vi "Test_Fitting.vi"() -> ()   [LabVIEW 2015]
panel:
  out "best fit parameters":dbl[](array[numeric])=[97.36526335937096, 65.50408984686088, 41.15888694388816, 22.4726351042886, 37.87775155788913]
  out "Generated Image":dbl[][](graph)
  out "error out":errorcluster
  out "Elapsed time in ms":u32=1425
  out "Best Fit":dbl[][](graph)
  in  "Image Size":cluster{"Width":dbl, "Height":dbl}={"Width"=100.0, "Height"=100.0}
  in  "Noise":dbl=10.0
  in  "Simulation":dbl[](array[slide])=[97.19626168224299, 65.42056074766354, 41.1214953271028, 22.429906542056074, 38.006230529595015, 104.04984423676012] caption="Amplitude\n\n\nX-Position\n\n\nY-Position\n\n\nWidth A\n\n\nWidth B\n\n\nAngle" scale=0.0..200.0
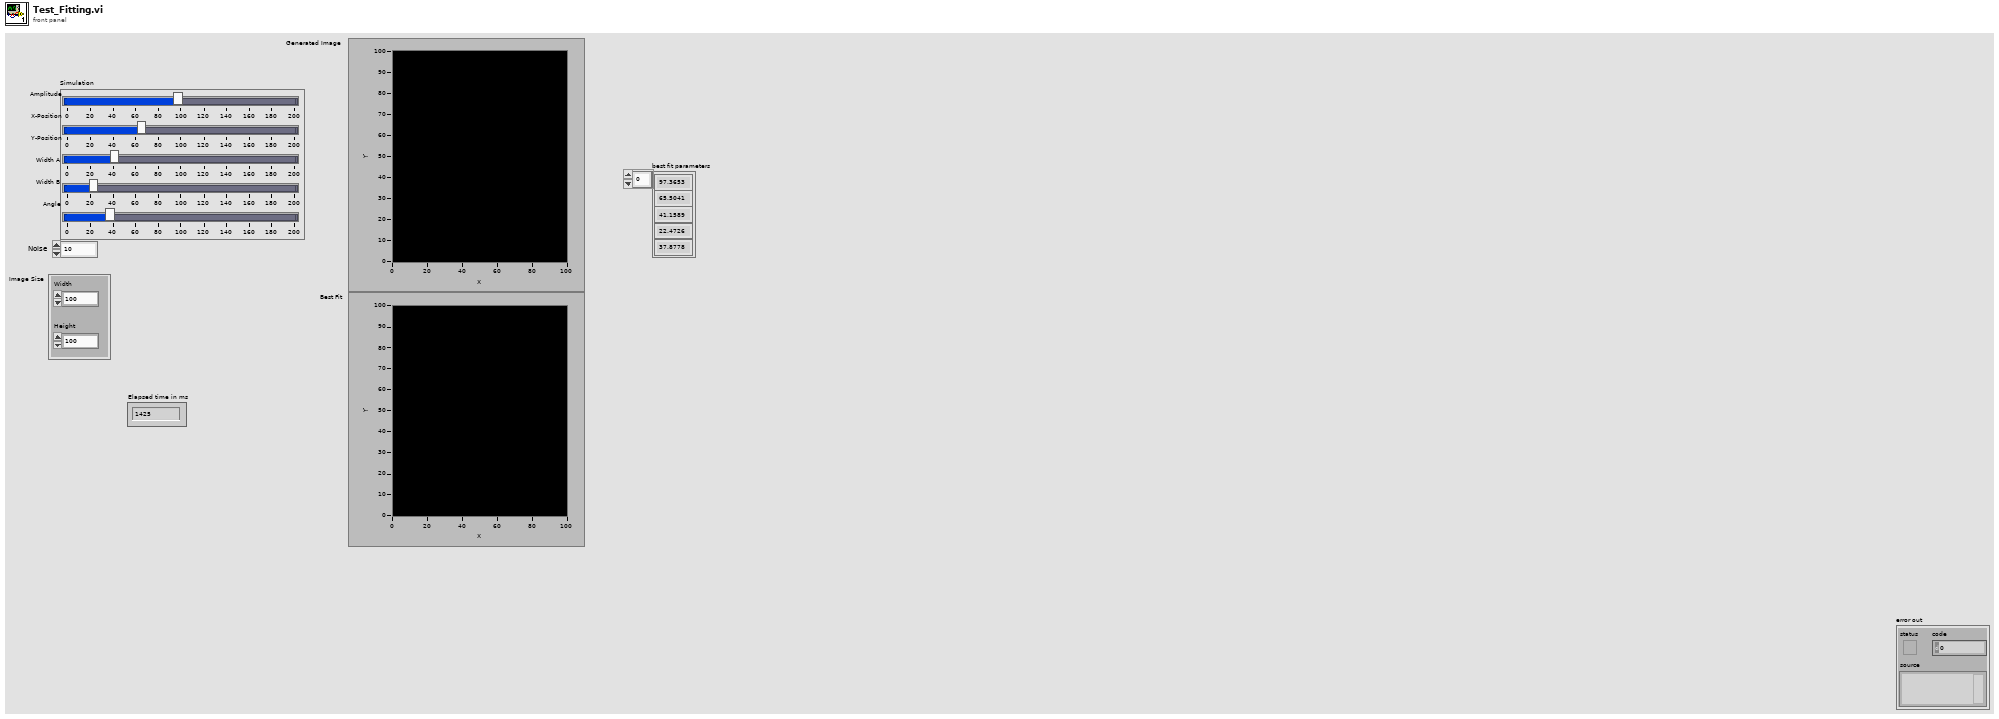
[diagram p1: front panel]
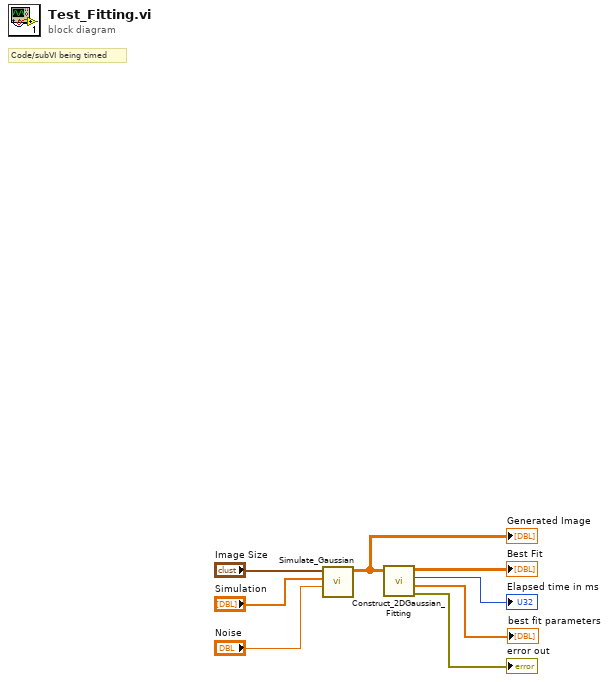
[diagram p0: block diagram]
diagram:
  # "Code/subVI being timed"
  n1 = call "Simulate_Gaussian.vi"("Noise"="Noise", "Simulation"="Simulation", "Sim Dim."="Image Size") -> ("OD(2D)"=w8:dbl[][])  [unwired: 8 in]
  "Generated Image" <- w8
  n2 = call "Construct_2DGaussian_Fitting.vi"("OD(2D)"=w8) -> ("error out"=→"error out":errorcluster, "best fit parameters"=→"best fit parameters":dbl[], "Elapsed time in ms"=→"Elapsed time in ms":u32, "Fit Image"=→"Best Fit":dbl[][])  [unwired: 7 in]
